vi "AlliGator Check Decay Pre-Processing Steps Needed.vi"(8 "Error In":errorcluster, 10 "Decay Preprocessing Parameters":T1={"Background Subtraction"=FALSE, "Straighten Decay"=FALSE, "Reverse Gates"=FALSE, "1-Normalized Decay"=FALSE, "Smoothen Decay"=FALSE, "Smoothing Parameter"=0.0, "Shift Decay"=FALSE, "Decay Shift Parameters"={"Type"=enum."Default", "Shift"=0.0, "Threshold"=0.0, "Rotate"=FALSE}, "Extrapolate Decay"=FALSE, "Additional Points"=0, "Head Fraction"=0.0, "Pixel-Normalize Decay"=FALSE, "Use Periodicity"=FALSE, "Use Cursors"=FALSE, "Tail Fraction"=0.0, "Use Decay Pre-Processing"=FALSE, "Fold Decay"=FALSE, "# Folds"=1, "[0-1]-Normalized Decay"=FALSE} {"# Folds" min=1}, 11 "Preprocessing Steps Order in":string[](array[string])) -> (0 "Error Out":errorcluster, 1 "Preprocessing needed?":bool, 2 "Decay Preprocessing Parameters (dup)":T1={"Background Subtraction"=FALSE, "Straighten Decay"=FALSE, "Reverse Gates"=FALSE, "1-Normalized Decay"=FALSE, "Smoothen Decay"=FALSE, "Smoothing Parameter"=0.0, "Shift Decay"=FALSE, "Decay Shift Parameters"={"Type"=enum."Default", "Shift"=0.0, "Threshold"=0.0, "Rotate"=FALSE}, "Extrapolate Decay"=FALSE, "Additional Points"=0, "Head Fraction"=0.0, "Pixel-Normalize Decay"=FALSE, "Use Periodicity"=FALSE, "Use Cursors"=FALSE, "Tail Fraction"=0.0, "Use Decay Pre-Processing"=FALSE, "Fold Decay"=FALSE, "# Folds"=1, "[0-1]-Normalized Decay"=FALSE} {"# Folds" min=1}, 3 "Preprocessing Steps Order out":string[](array[string]), 4 "Message":string)   [LabVIEW 2021, in "AlliGator Phasor Plot.lvlib"]
doc: "Checks whether any decay pre-processing is needed."
uses:
  AlliGator Phasor Plot.lvlib
  Decay Analysis/Decay Preprocessing/AlliGator Decay Preprocessing Parameters.ctl
  Graphs/XY Graph/XY Graph Plot Shift Parameters.ctl
  Graphs/XY Graph/XY Graph Plot Shift Method.ctl
  Variant/Variant.lvlib
  Strings/Strings.lvlib
  Graphs/XY Graph/XY Graph Add-Ons.lvlib
  Decay Analysis/Decay Preprocessing/AlliGator Decay Preprocessing.lvlib
panel:
  # "see the AlliGator License on the block diagram (Ctrl+E or Window:Show Block Diagram)"
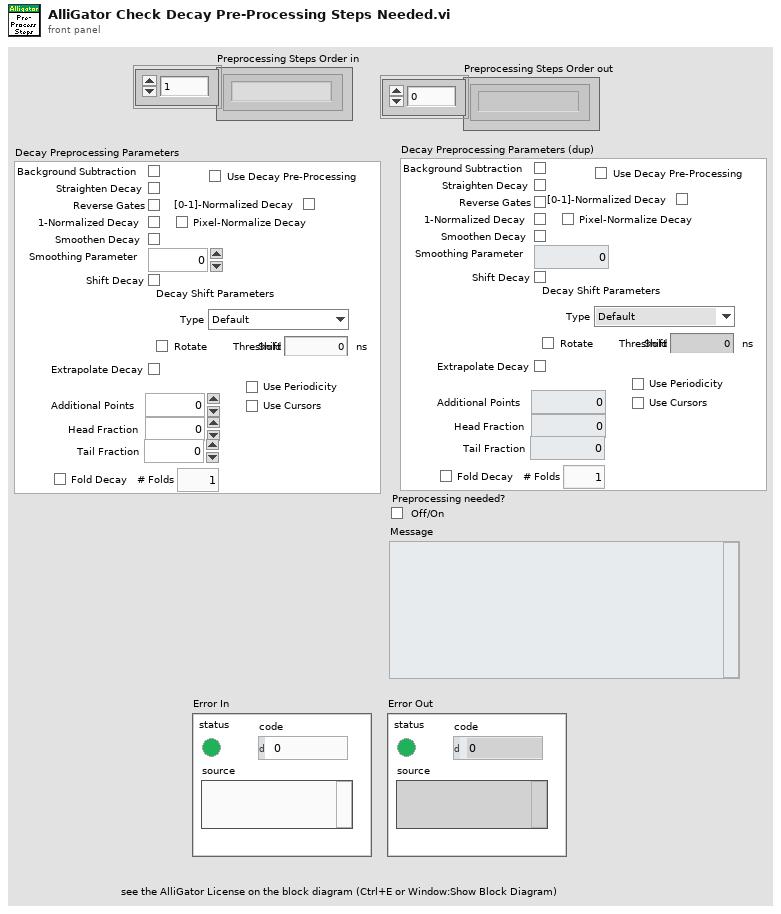
[diagram p1: front panel]
types:
  T1 = typedef "AlliGator Decay Preprocessing.lvlib/AlliGator Decay Preprocessing Parameters.ctl" = cluster{"Background Subtraction":bool, "Straighten Decay":bool, "Reverse Gates":bool, "1-Normalized Decay":bool, "Smoothen Decay":bool, "Smoothing Parameter":dbl, "Shift Decay":bool, "Decay Shift Parameters":T2, "Extrapolate Decay":bool, "Additional Points":u32, "Head Fraction":dbl, "Pixel-Normalize Decay":bool, "Use Periodicity":bool, "Use Cursors":bool, "Tail Fraction":dbl, "Use Decay Pre-Processing":bool, "Fold Decay":bool, "# Folds":u32, "[0-1]-Normalized Decay":bool}
  T2 = typedef "XY Graph Add-Ons.lvlib/XY Graph Plot Shift Parameters.ctl" = cluster{"Type":T3, "Shift":dbl[unit], "Threshold":dbl, "Rotate":bool}
  T3 = typedef "XY Graph Add-Ons.lvlib/XY Graph Plot Shift Method.ctl" = enum16{"Default", "CFD", "Threshold", "Cross-Correlation"}
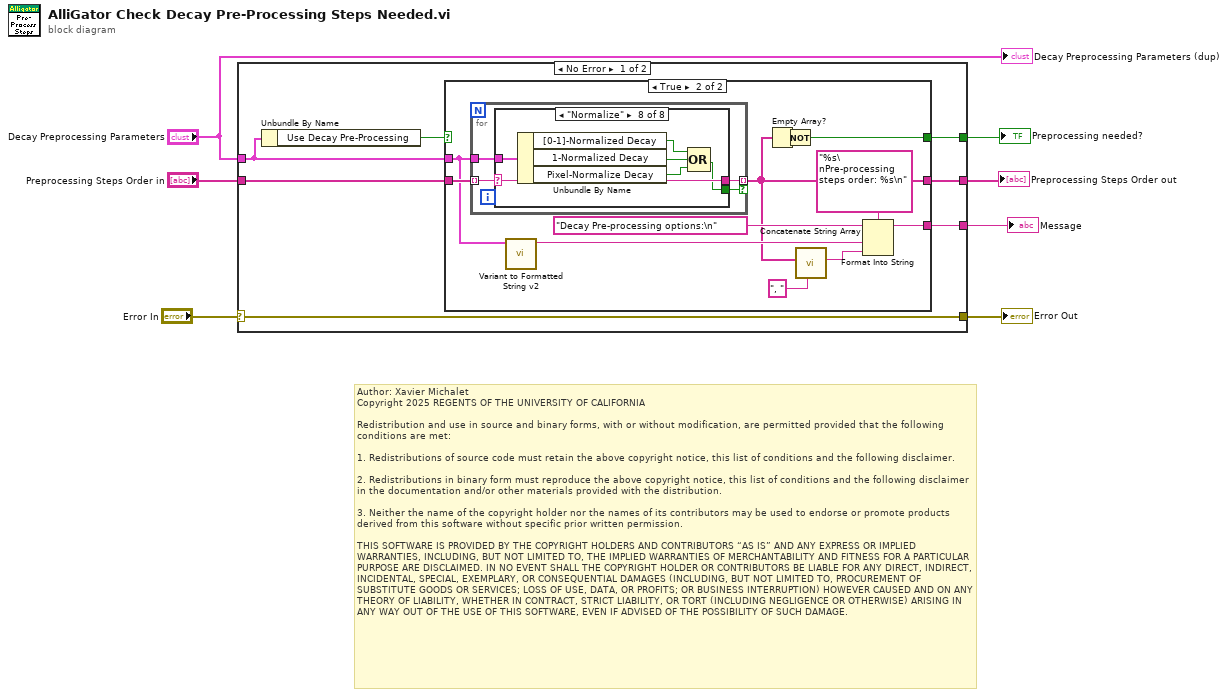
[diagram p0: block diagram]
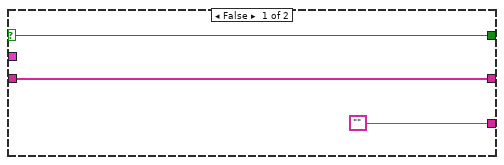
[diagram p2: hidden frame]
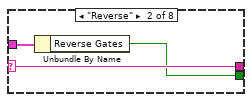
[diagram p4: hidden frame]
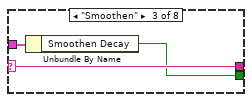
[diagram p5: hidden frame]
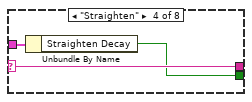
[diagram p6: hidden frame]
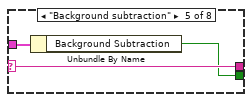
[diagram p7: hidden frame]
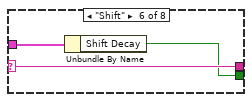
[diagram p8: hidden frame]
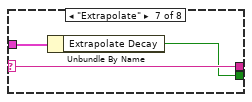
[diagram p9: hidden frame]
diagram:
  # "Author: Xavier Michalet\nCopyright 2025 REGENTS OF THE UNIVERSITY OF CALIFORNIA\n\nRedistribution and use in source and binary forms, with or without modification, are permitted provided that the following conditions are met:\n\n1. Redistributions of source code must retain the above copyright notice, this list of conditions and the following disclaimer.\n\n2. Redistributions in binary form must reproduce the above copyright notice, this list of conditions and the following disclaimer in the documentation and/or other materials provided with the distribution.\n\n3. Neither the name of the copyright holder nor the names of its contributors may be used to endorse or promote products derived from this software without specific prior written permission.\n\nTHIS SOFTWARE IS PROVIDED BY THE COPYRIGHT HOLDERS AND CONTRIBUTORS “AS IS” AND ANY EXPRESS OR IMPLIED WARRANTIES, INCLUDING, BUT NOT LIMITED TO, THE IMPLIED WARRANTIES OF MERCHANTABILITY AND FITNESS FOR A PARTICULAR PURPOSE ARE DISCLAIMED. IN NO EVENT SHALL THE COPYRIGHT HOLDER OR CONTRIBUTORS BE LIABLE FOR ANY DIRECT, INDIRECT, INCIDENTAL, SPECIAL, EXEMPLARY, OR CONSEQUENTIAL DAMAGES (INCLUDING, BUT NOT LIMITED TO, PROCUREMENT OF SUBSTITUTE GOODS OR SERVICES; LOSS OF USE, DATA, OR PROFITS; OR BUSINESS INTERRUPTION) HOWEVER CAUSED AND ON ANY THEORY OF LIABILITY, WHETHER IN CONTRACT, STRICT LIABILITY, OR TORT (INCLUDING NEGLIGENCE OR OTHERWISE) ARISING IN ANY WAY OUT OF THE USE OF THIS SOFTWARE, EVEN IF ADVISED OF THE POSSIBILITY OF SUCH DAMAGE."
  n1 = case shown="No Error" "Error In" {
    selector: "Error In" -> [w10 w58]
    tunnel: [w13 _] -> w7
    tunnel: "Preprocessing Steps Order in" -> [w12 w57]
    tunnel: [w11 w57] -> w5
    tunnel: "Decay Preprocessing Parameters" -> [w9 _]
    tunnel: [w10 w58] -> w2
    tunnel: [w8 _] -> w1
    frame No Error {
      n2 = Unbundle By Name(w9) -> ("Use Decay Pre-Processing"=w14:bool)
      n3 = case shown="True" w14 {
        selector: w14 -> [w17 _]
        tunnel: [w17 w26] -> w13
        tunnel: w12 -> [w16 w28]
        tunnel: w9 -> [_ w24]
        tunnel: [w16 w20] -> w11
        tunnel: ["" w25] -> w8
        frame False {
        }
        frame True {
          n4 = for {
            tunnel: w28 -> [w32] mode=indexing
            tunnel: w24 -> [w31]
            tunnel: [w30] -> w20 mode=indexing if=w29
            n5 = case shown="\"Normalize\"" w32 {
              selector: w32 -> [_ w34 w37 w40 w43 w46 w49 w55]
              tunnel: w31 -> [_ w35 w38 w41 w44 w47 w50 w56]
              tunnel: [_ w34 w37 w40 w43 w46 w49 w55] -> w30
              tunnel: [_ w33 w36 w39 w42 w45 w48 w53] -> w29
              frame "", Default {
              }
              frame "Reverse" {
                n6 = Unbundle By Name(w35) -> ("Reverse Gates"=w33:bool)
              }
              frame "Smoothen" {
                n7 = Unbundle By Name(w38) -> ("Smoothen Decay"=w36:bool)
              }
              frame "Straighten" {
                n8 = Unbundle By Name(w41) -> ("Straighten Decay"=w39:bool)
              }
              frame "Background subtraction" {
                n9 = Unbundle By Name(w44) -> ("Background Subtraction"=w42:bool)
              }
              frame "Shift" {
                n10 = Unbundle By Name(w47) -> ("Shift Decay"=w45:bool)
              }
              frame "Extrapolate" {
                n11 = Unbundle By Name(w50) -> ("Extrapolate Decay"=w48:bool)
              }
              frame "Normalize" {
                n12 = Unbundle By Name(w56) -> ("[0-1]-Normalized Decay"=w51:bool, "1-Normalized Decay"=w54:bool, "Pixel-Normalize Decay"=w52:bool)
                n13 = Compound Arithmetic op=OR(w51, w54, w52) -> (w53:bool)
              }
            }
          }
          n14 = call "Variant to Formatted String v2.vi"("Anything"=w24) -> ("String"=w23:string)  [unwired: 9 in, 1 out]
          n15 = Empty Array?(array=w20) -> (empty?=w27:bool)
          n16 = Not(x=w27) -> (.not. x?=w26:bool)
          n17 = call "Concatenate String Array.vi"("Separator (TAB)"=", ", "String Array"=w20) -> ("Formatted String"=w18:string)  [unwired: 9 in]
          n18 = Format Into String(format string="%s\nPre-processing steps order: %s\n", initial string="Decay Pre-processing options:\n", w23, w18) -> (resulting string=w25:string)  [unwired: 1 in, 1 out]
        }
      }
    }
    frame Error {
    }
  }
  "Preprocessing needed?" <- w7
  "Preprocessing Steps Order out" <- w5
  "Message" <- w1
  "Error Out" <- w2
  "Decay Preprocessing Parameters (dup)" <- "Decay Preprocessing Parameters"
